vi "Vector.vi"() -> ()   [LabVIEW 2017, in "Examples.lvlib"]
uses:
  Examples.lvlib
panel:
  out "Waveform Chart F401013 - F401011":sgl(graph)
  out "Waveform Chart F401011 + F401013":sgl(graph)
  out "x-y":sgl
  out "x+y":sgl
  out "Error Out 401015":errorcluster
  out "Waveform Chart F401015":sgl(graph)
  out "F401015":sgl
  out "Waveform Chart F401013":sgl(graph)
  out "Waveform Chart F401011":sgl(graph)
  out "Waveform Chart F401009":sgl(graph)
  out "Waveform Chart F401007":sgl(graph)
  out "Waveform Chart 401001":i64(graph)
  out "Error Out F401013":errorcluster
  out "F401013":sgl
  out "Error Out F401011":errorcluster
  out "F401011":sgl
  out "Error Out F401009":errorcluster
  out "F401009":sgl
  out "Error Out F401007":errorcluster
  out "F401007":sgl
  out "Error Out 401001":errorcluster
  out "401001":i64
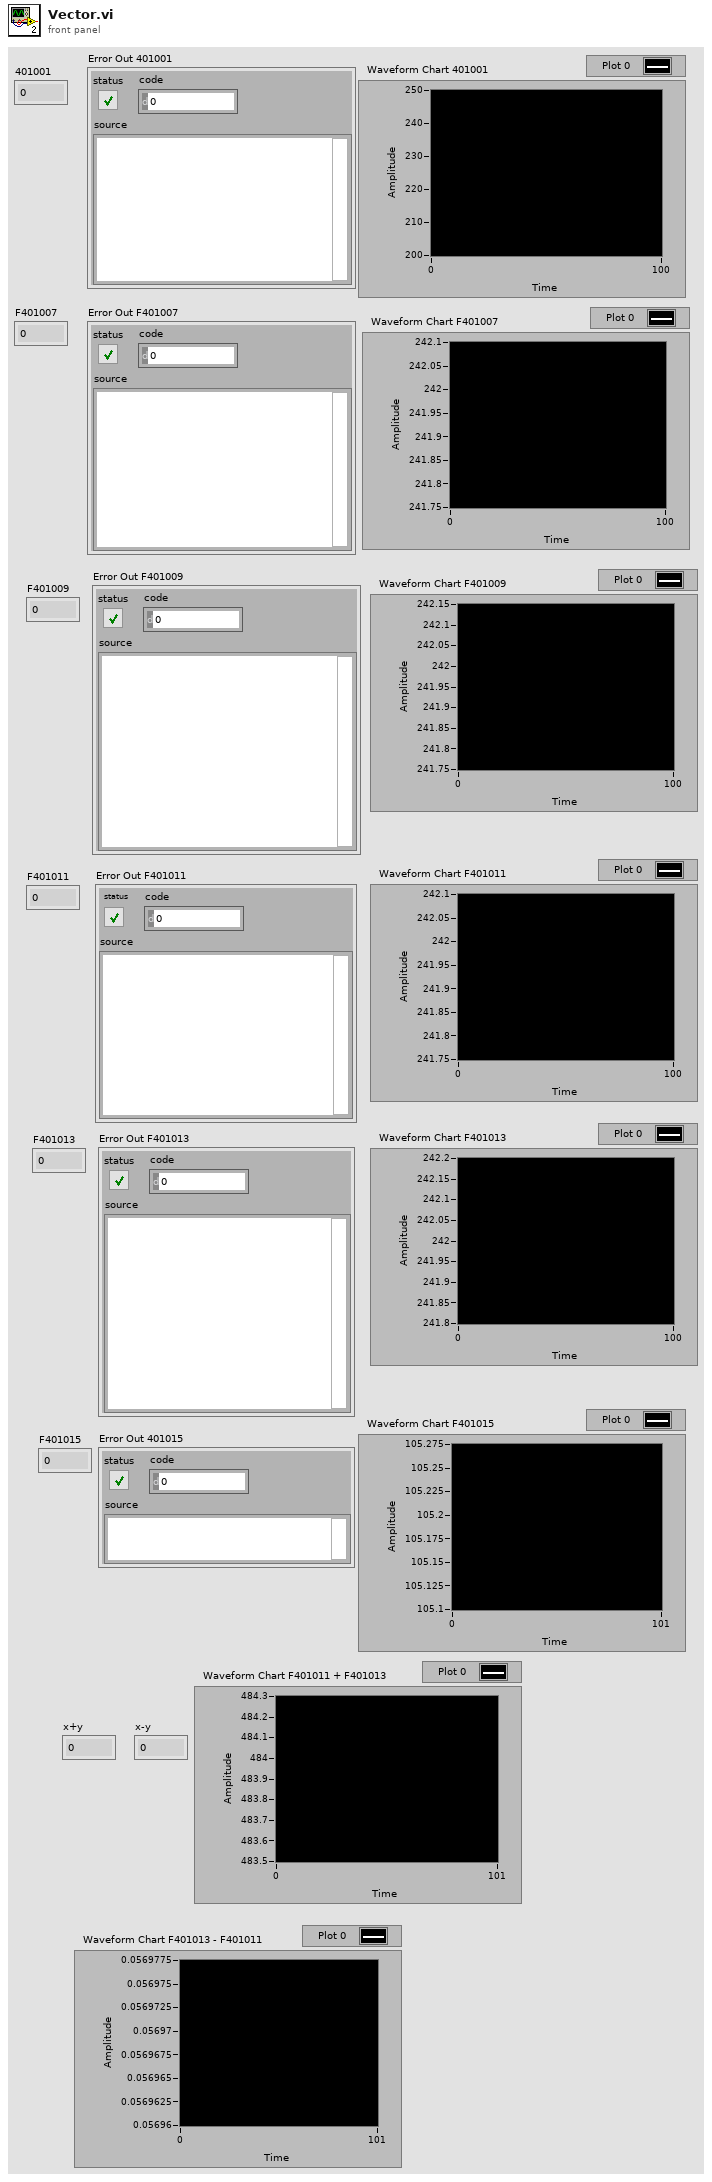
[diagram p1: front panel]
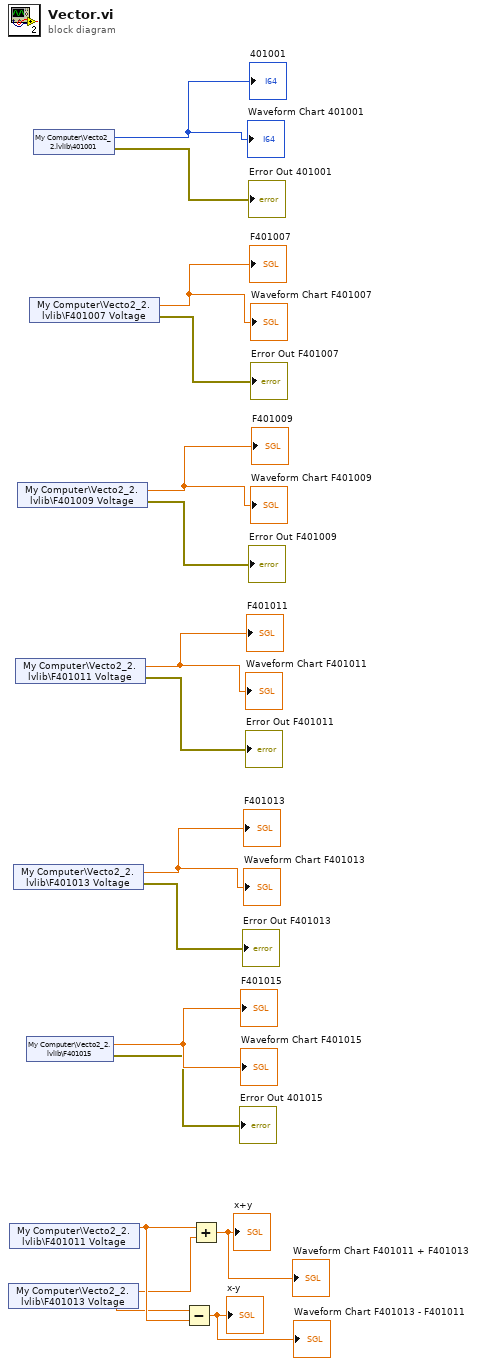
[diagram p0: block diagram]
diagram:
  n1 = shared-variable "My Computer\\Vecto2_2.lvlib\\F401013 Voltage"() -> (w3:sgl)  [unwired: 1 in, 1 out]
  n2 = shared-variable "My Computer\\Vecto2_2.lvlib\\F401011 Voltage"() -> (w4:sgl)  [unwired: 1 in, 1 out]
  n3 = shared-variable "My Computer\\Vecto2_2.lvlib\\F401013 Voltage"() -> (→"F401013" →"Waveform Chart F401013":sgl, error out=→"Error Out F401013":errorcluster)  [unwired: 1 in]
  n4 = shared-variable "My Computer\\Vecto2_2.lvlib\\F401011 Voltage"() -> (→"F401011" →"Waveform Chart F401011":sgl, error out=→"Error Out F401011":errorcluster)  [unwired: 1 in]
  n5 = shared-variable "My Computer\\Vecto2_2.lvlib\\F401009 Voltage"() -> (→"F401009" →"Waveform Chart F401009":sgl, error out=→"Error Out F401009":errorcluster)  [unwired: 1 in]
  n6 = shared-variable "My Computer\\Vecto2_2.lvlib\\F401015"() -> (→"F401015" →"Waveform Chart F401015":sgl, error out=→"Error Out 401015":errorcluster)  [unwired: 1 in]
  n7 = shared-variable "My Computer\\Vecto2_2.lvlib\\F401007 Voltage"() -> (→"F401007" →"Waveform Chart F401007":sgl, error out=→"Error Out F401007":errorcluster)  [unwired: 1 in]
  n8 = shared-variable "My Computer\\Vecto2_2.lvlib\\401001"() -> (→"401001" →"Waveform Chart 401001":i64, error out=→"Error Out 401001":errorcluster)  [unwired: 1 in]
  n9 = Subtract(x=w3, y=w4) -> (x-y=→"x-y" →"Waveform Chart F401013 - F401011":sgl)
  n10 = Add(x=w4, y=w3) -> (x+y=→"x+y" →"Waveform Chart F401011 + F401013":sgl)
